vi "emergency abort VI.vi"() -> ()   [LabVIEW 2009]
panel:
  out "error out":errorcluster
  in  "error in (no error)":errorcluster
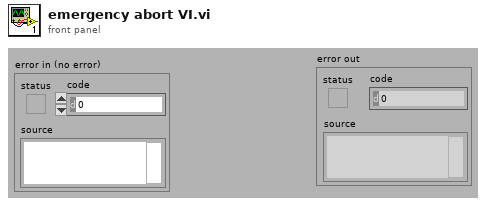
[diagram p1: front panel]
types:
  T1 = enum32{"Bad", "Idle", "Run top level", "Running"}
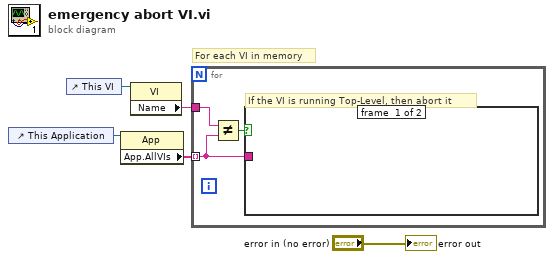
[diagram p0: block diagram]
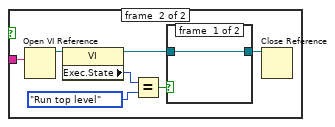
[diagram p2: hidden frame]
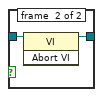
[diagram p3: hidden frame]
diagram:
  # "For each VI in memory"
  n1 = control-ref of="This Application"() -> (w3:refnum<vi>)
  n2 = control-ref of="This VI"() -> (w4:refnum<vi>)
  n3 = property class="App"(reference=w3) -> ("App.AllVIs"=w1:string[])  [unwired: 1 in, 2 out]
  n4 = property class="VI"(reference=w4) -> ("Name"=w2:string)  [unwired: 1 in, 2 out]
  n5 = for {
    tunnel: w2 -> [w8]
    tunnel: w1 -> [w6] mode=indexing
    # "If the VI is running Top-Level, then abort it"
    n6 = Not Equal?(x=w8, y=w6) -> (x != y?=w7:bool)
    n7 = case shown="True" w7 {
      tunnel: w6 -> [_ w15]
      frame #0 {
      }
      frame #1 {
        n8 = Open VI Reference(vi path=w15) -> (vi reference=w14:refnum<vi>)  [unwired: 5 in, 1 out]
        n9 = property class="VI"(reference=w14) -> (reference out=w10:refnum<vi>, "Exec.State"=w13:T1)  [unwired: 1 in, 1 out]
        n10 = Equal?(x=w13, y=T1."Run top level" ("Execution:State")) -> (x = y?=w11:bool)
        n11 = case shown="False" w11 {
          tunnel: w10 -> [w16 w18]
          tunnel: [w16 w17] -> w9
          frame #0 {
          }
          frame #1 {
            n12 = invoke class="VI" method="Abort VI"(reference=w18) -> (reference out=w17:refnum<vi>)  [unwired: 2 in, 2 out]
          }
        }
        n13 = Close Reference(reference=w9) -> ()  [unwired: 1 in, 1 out]
      }
    }
  }
  "error out" <- "error in (no error)"
